vi "Perform I2C Test.vi"(8 "error in (no error)":errorcluster, 11 "LCM Single-Up MTS Test in":refnum<class "LCM Single-Up MTS Test.lvclass">) -> (0 "error out":errorcluster, 3 "I2C Data Match":bool)   [LabVIEW 2015, in "LCM Single-Up MTS Test.lvclass"]
uses:
  LCM Single-Up MTS Test.lvclass
  <vilib>/Cree, Inc/Cree Test Framework/Core Launcher/Core Manager Methods -- Enum.ctl
  Classes/Instruments/I2C Device/NI-8452/Public API/Slave Wait on Event.vi
  Classes/Manufacturing Test/Class/SC Manufacturing Test.lvclass
  Classes/Instruments/I2C Device/NI-8452/NI-8452.lvclass
  <vilib>/Cree, Inc/Cree Test Framework/Classes/Base Objects/Base Class/Base Class/Base Class.lvclass
  <vilib>/Cree, Inc/Cree Test Framework/Core Launcher/Core Launcher.lvlib
  <vilib>/Cree, Inc/Cree Test Framework/Classes/Data/Data Repo/Class/Data Repo.lvclass
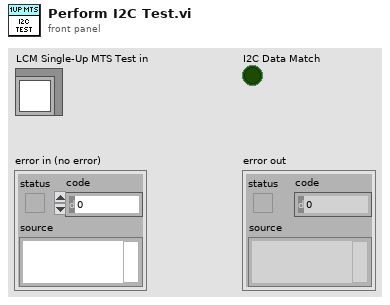
[diagram p1: front panel]
types:
  T1 = typedef "Core Launcher.lvlib/Core Manager Methods -- Enum.ctl" = enum16{"Spawn Objects", "Get Objects", "Destroy Objects"}
  T2 = typedef "ni845xI2cSlaveEventType.ctl" = enum8{"NoEvent", "CmdEvent", "DataAvailEvent", "DataReqEvent", "WriteCompleteEvent"}
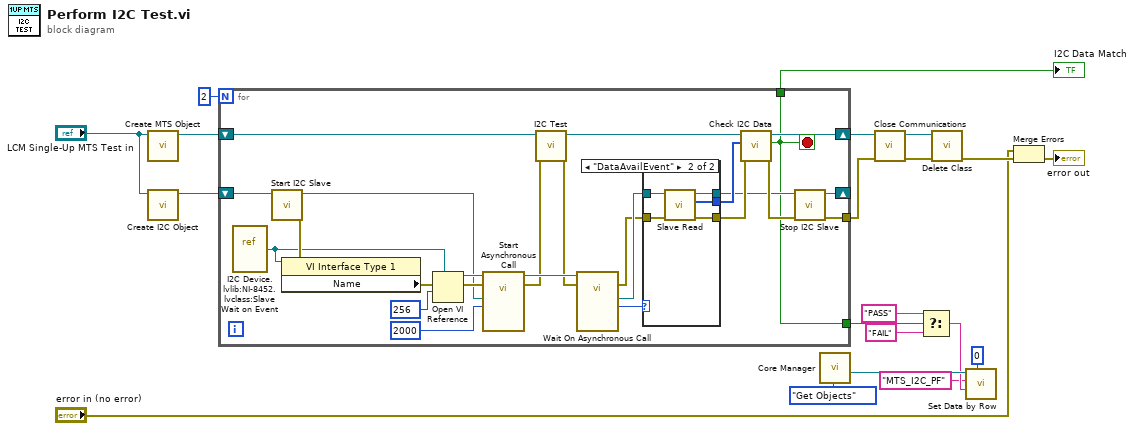
[diagram p0: block diagram]
diagram:
  n1 = call "Create MTS Object.vi"("LCM Single-Up MTS Test in"="LCM Single-Up MTS Test in") -> ("MTS"=w7:refnum<class "SC Manufacturing Test.lvclass">)  [unwired: 9 in, 1 out]
  n2 = call "Create I2C Object.vi"("LCM Single-Up MTS Test in"="LCM Single-Up MTS Test in") -> ("I2C"=w5:refnum<class "NI-8452.lvclass">)  [unwired: 9 in, 1 out]
  n3 = for {
    N: 2 -> [_]
    shift-right: [w27] -> w4
    shift-left: w7 -> [w42]
    shift-right: [w22] -> _
    shift-left: w5 -> [w43]
    tunnel: [w21] -> w19
    tunnel: [w21] -> w8
    tunnel: [w24] -> w3
    stop <- w21 stop-if-true
    n4 = vi-ref "I2C Device.lvlib:NI-8452.lvclass:Slave Wait on Event.vi"() -> (w41:refnum<vi>)
    n5 = call "Start I2C Slave.vi"("NI-8452 in"=w43) -> ("error out"=w44:errorcluster, "NI-8452 out"=w38:refnum<class "NI-8452.lvclass">)  [unwired: 9 in]
    n6 = property class="VI Interface Type 1"(reference=w41) -> ("Name"=w40:string)  [unwired: 1 in, 2 out]
    n7 = Open VI Reference(type specifier VI Refnum (for type only)=w41, vi path=w40, options=256) -> (vi reference=w39:refnum<vi>)  [unwired: 3 in, 1 out]
    n8 = call-by-ref "Start Asynchronous Call"(reference=w39, error in=w44, "Timeout (500ms)"=u32 2000, "NI-8452 in"=w38) -> (reference out=w36:refnum<vi>, error out=w35:errorcluster)  [unwired: 6 in, 4 out]
    n9 = call "I2C Test.vi"("error in (no error)"=w35, "Acrobat Template in"=w42) -> ("error out"=w34:errorcluster, "Acrobat Template out"=w30:refnum<class "SC Manufacturing Test.lvclass">)  [unwired: 8 in]
    n10 = call-by-ref "Wait On Asynchronous Call"(reference=w36, error in=w34) -> (error out=w32:errorcluster, "Event Type"=w31:T2, "NI-8452 out"=w33:refnum<class "NI-8452.lvclass">)  [unwired: 8 in, 3 out]
    n11 = case shown="\"DataAvailEvent\"" w31 {
      tunnel: w33 -> [w46 w51]
      tunnel: w32 -> [w45 w50]
      tunnel: [w46 w49] -> w23
      tunnel: [w45 w48] -> w28
      tunnel: [_ w47] -> w29
      frame Default {
      }
      frame "DataAvailEvent" {
        n12 = call "Slave Read.vi"("error in (no error)"=w50, "NI-8452 in"=w51) -> ("error out"=w48:errorcluster, "Data"=w47:u8[], "NI-8452 out"=w49:refnum<class "NI-8452.lvclass">)  [unwired: 7 in]
      }
    }
    n13 = call "Check I2C Data.vi"("error in (no error)"=w28, "Data"=w29, "Acrobat Template in"=w30) -> ("error out"=w25:errorcluster, "I2C Data Match"=w21:bool, "Acrobat Template out"=w27:refnum<class "SC Manufacturing Test.lvclass">)  [unwired: 6 in]
    n14 = call "Stop I2C Slave.vi"("error in (no error)"=w25, "NI-8452 in"=w23) -> ("error out"=w24:errorcluster, "NI-8452 out"=w22:refnum<class "NI-8452.lvclass">)  [unwired: 8 in]
  }
  "I2C Data Match" <- w8
  n15 = call <vilib>:"Core Manager.vi"("Method"=Core_Manager_Methods_--_Enum."Get Objects") -> ("Data Repo"=w18:refnum<class "Data Repo.lvclass">)  [unwired: 7 in, 3 out]
  n16 = call "Close Communications.vi"("error in (no error)"=w3, "Acrobat Template in"=w4) -> ("error out"=w2:errorcluster, "Acrobat Template out"=w1:refnum<class "SC Manufacturing Test.lvclass">)  [unwired: 8 in]
  n17 = Select(t="PASS" ("Header"), s=w19, f="FAIL" ("Header")) -> (s? t:f=w15:string)
  n18 = call <vilib>:"Delete Class.vi"("error in (no error)"=w2, "Base Class in"=w1) -> ("error out"=w11:errorcluster)  [unwired: 8 in, 1 out]
  n19 = call <vilib>:"Set Data by Row.vi"("Row"=0, "Value"=w15, "Header"="MTS_I2C_PF", "Acrobat Template in"=w18) -> ()  [unwired: 6 in, 2 out]
  n20 = Merge Errors("error in (no error)", w11) -> (→"error out":errorcluster)
